vi "Day 14-Build Polymer Map.vi"(11 "Polymer Input":string[](array[string])) -> (3 "Polymer Template Map":map{string, string}(c390))   [LabVIEW 2021]
uses:
  <vilib>/regexp/Match Regular Expression.xnode
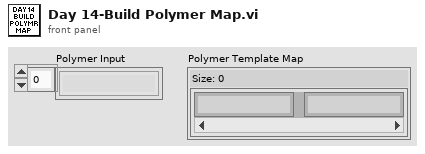
[diagram p1: front panel]
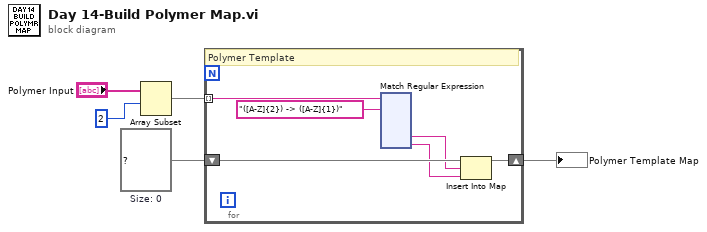
[diagram p0: block diagram]
diagram:
  w4 = map{string, string} {}  # Size: 0
  n1 = Array Subset(array="Polymer Input", index=2) -> (w2:string[])  [unwired: 1 in]
  n2 = for {
    tunnel: w2 -> [w11] mode=indexing
    shift-right: [w9] -> w5
    shift-left: w4 -> [w8]
    # "Polymer Template"
    n3 = xnode "Match Regular Expression"("input string"=w11, "regular expression"="([A-Z]{2}) -> ([A-Z]{1})") -> ("submatch 1"=w7:string, "submatch 2"=w6:string)  [unwired: 4 in, 5 out]
    n4 = Insert Into Map(map in=w8, key=w7, value=w6) -> (map out=w9:map{string, string})  [unwired: 2 out]
  }
  "Polymer Template Map" <- w5
